vi "uObserver_Publish_Event_Blocking_Reply.vi"(6 "timeout in ms (2000)":i32=2000, 8 "error in (no error)":errorcluster, 9 "data":refnum<class "uData.lvclass">, 10 "command":string, 11 "uObserver in":refnum<class "uObserver.lvclass">) -> (0 "error out":errorcluster, 1 "reply":refnum<class "uData.lvclass">, 3 "uObserver out":refnum<class "uObserver.lvclass">)   [LabVIEW 2021, in "uFramework_pack_uActor.lvlib" / "uObserver.lvclass"]
doc: "Publish an event to the observed broker conforming to the Observer's publishing policy and block data flow until a reply is received.\n\nUse sparsely due to risk of dead locks, risk of multiple receipients all sending replies and risk of no listener replying.\n\nThis method returns error 550011 on error."
uses:
  uObserver.lvclass
  uObserver.lvclass/uObserver.ctl
  Bin/uFramework.lvlibp/uTransport_Queue/uTransport_Queue.lvclass
  Bin/uFramework.lvlibp/uMsg/uMsg.lvclass
  <vilib>/Utility/error.llb/Error Cluster From Error Code.vi
  <vilib>/ErrorRing/Error Ring.xnode
  U:/Projects/uFramework/Bin/uFramework.lvlibp/uTransport_Queue/uTransport_Queue.lvclass
  U:/Projects/uFramework/Bin/uFramework.lvlibp/uTransport/uTransport.lvclass
  Bin/uData.lvlibp/uData.lvclass
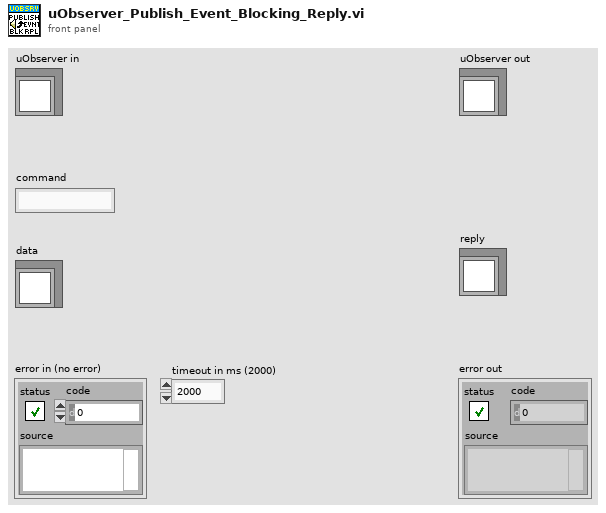
[diagram p1: front panel]
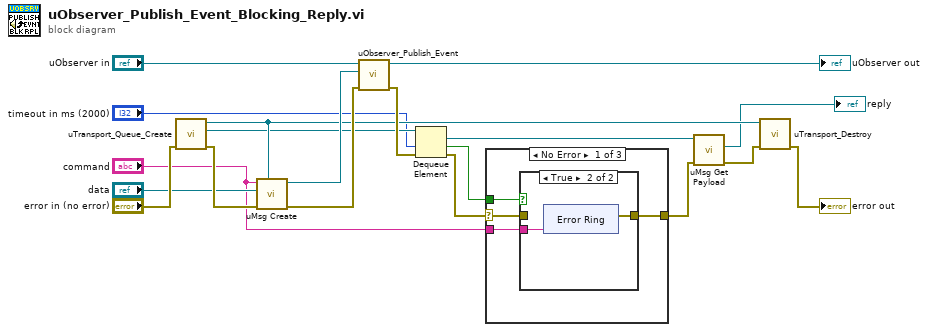
[diagram p0: block diagram]
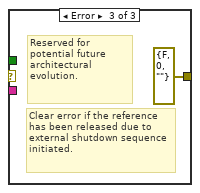
[diagram p4: hidden frame]
diagram:
  n1 = call "uTransport_Queue_Create.vi"("error in (no error)"="error in (no error)") -> ("error out"=w15:errorcluster, "queue"=w9:refnum<queue>, "uTransport_Queue out"=w11:refnum<class "uTransport_Queue.lvclass">)  [unwired: 8 in]
  n2 = call "uMsg Create.vi"("Reply Transport"=w11, "error in (no error)"=w15, "Payload"="data", "CMD"="command") -> ("error out"=w13:errorcluster, "uMsg out"=w14:refnum<class "uMsg.lvclass">)  [unwired: 6 in]
  n3 = call "uObserver_Publish_Event.vi"("error in (no error)"=w13, "uMsg"=w14, "uObserver in"="uObserver in") -> ("error out"=w19:errorcluster, "uObserver out"=→"uObserver out":refnum<class "uObserver.lvclass">)  [unwired: 7 in]
  n4 = Dequeue Element(queue=w9, timeout in ms (-1)="timeout in ms (2000)", error in (no error)=w19) -> (element=w5:refnum<class "uMsg.lvclass">, timed out?=w1:bool, error out=w7:errorcluster)  [unwired: 1 out]
  n5 = case shown="No Error" w7 {
    selector: w7 -> [w20 w34 _]
    tunnel: [w22 w34 errorcluster {"status"=FALSE, "code"=0, "source"=""} ("error IO")] -> w3
    tunnel: "command" -> [w23 _ _]
    tunnel: w1 -> [w21 _ _]
    frame No Error {
      n6 = case shown="True" w21 {
        tunnel: w23 -> [_ w26]
        tunnel: [w24 w25] -> w22
        tunnel: w20 -> [w24 _]
        frame False {
        }
        frame True {
          n7 = xnode "Error Ring"("parameter 0"=w26) -> ("error out"=w25:errorcluster)
        }
      }
    }
    frame Default {
    }
    frame Error {
      # "Reserved for potential future architectural evolution."
      # "Clear error if the reference has been released due to external shutdown sequence initiated."
    }
  }
  n8 = call "uMsg Get Payload.vi"("error in (no error)"=w3, "uMsg in"=w5) -> ("error out"=w6:errorcluster, "uData"=→"reply":refnum<class "uData.lvclass">)  [unwired: 7 in, 1 out]
  n9 = call-dynamic "uTransport_Destroy.vi"("error in (no error)"=w6, "uTransport_Queue in"=w11) -> ("error out"=→"error out":errorcluster)  [unwired: 9 in]
